vi "close_hw.vi"(8 "error in (no error)":errorcluster, 11 "ESP301viaTCPIP in":refnum<class "ESP301viaTCPIP.lvclass">) -> (0 "error out":errorcluster, 3 "ESP301viaTCPIP out":refnum<class "ESP301viaTCPIP.lvclass">)   [LabVIEW 2019, in "ESP301viaTCPIP.lvlib" / "ESP301viaTCPIP.lvclass"]
uses:
  ESP301viaTCPIP.lvclass
  ESP301viaTCPIP.lvlib
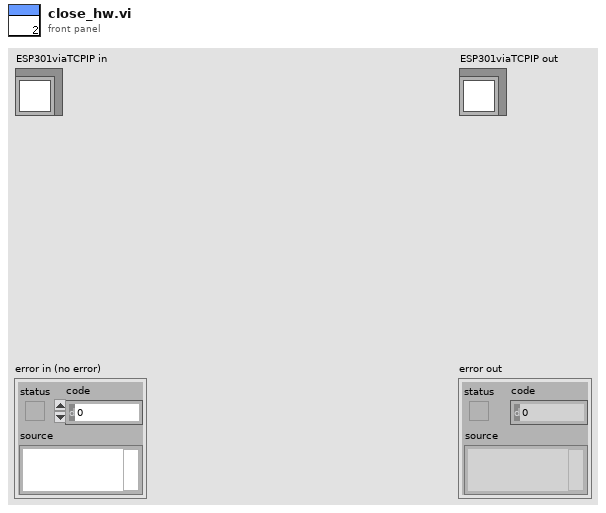
[diagram p1: front panel]
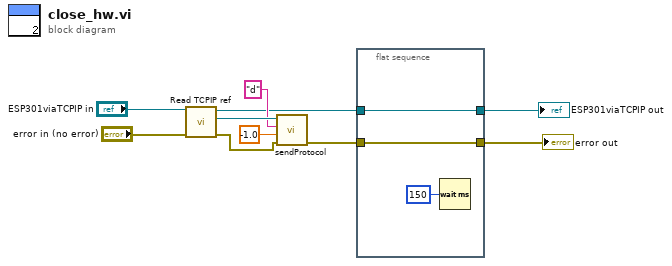
[diagram p0: block diagram]
diagram:
  n1 = call-dynamic "Read TCPIP ref.vi"("error in (no error)"="error in (no error)", "ESP301viaTCPIP in"="ESP301viaTCPIP in") -> ("error out"=w5:errorcluster, "TCPIP ref"=w8:refnum<k5>, "ESP301viaTCPIP out"=w1:refnum<class "ESP301viaTCPIP.lvclass">)  [unwired: 7 in]
  n2 = call "sendProtocol.vi"("error in (no error)"=w5, "GoTo position"=-1.0, "command"="d", "TCP Network Connection in"=w8) -> ("error out"=w3:errorcluster)  [unwired: 6 in, 1 out]
  n3 = flat-sequence {
    tunnel: [w13] -> w4
    tunnel: w3 -> [w13]
    tunnel: [w12] -> w2
    tunnel: w1 -> [w12]
    frame #0 {
      n4 = Wait (ms)(milliseconds to wait=u32 150) -> ()  [unwired: 1 out]
    }
  }
  "error out" <- w4
  "ESP301viaTCPIP out" <- w2
